vi "save program.vi"(8 "error in (no error)":errorcluster, 10 "Array":T1=[{"Action"=enum."Start", "Angle Min [°]"=0.0, "Angle Max [°]"=0.0, "Torque Min [oz-in]"=0.0, "Torque Max [oz-in]"=0.0}, {"Action"=enum."Return to Home", "Angle Min [°]"=0.0, "Angle Max [°]"=0.0, "Torque Min [oz-in]"=0.0, "Torque Max [oz-in]"=0.0}, {"Action"=enum."End", "Angle Min [°]"=0.0, "Angle Max [°]"=0.0, "Torque Min [oz-in]"=0.0, "Torque Max [oz-in]"=0.0}], 11 "Programs in":refnum<class "Programs.lvclass">) -> (0 "error out":errorcluster, 3 "Programs out":refnum<class "Programs.lvclass">)   [LabVIEW 2025, in "Programs.lvclass"]
uses:
  Programs.lvclass
  Programs.lvclass/Programs.ctl
  <vilib>/JDP Science/JSONtext/JSONtext.lvlib
  Controls/Sequencer/action enum.ctl
  Controls/Sequencer/step cluster.ctl
  Controls/Sequencer/sequence array.ctl
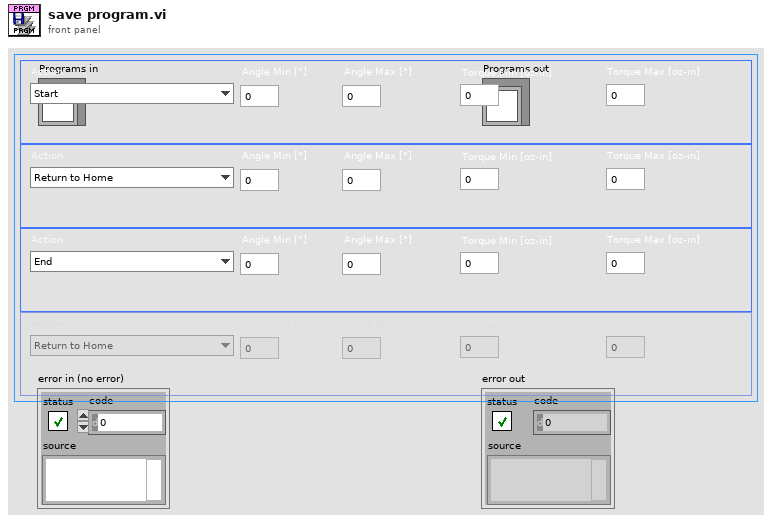
[diagram p1: front panel]
types:
  T1 = typedef "sequence array.ctl" = T2[]
  T2 = typedef "step cluster.ctl" = cluster{"Action":T3, "Angle Min [°]":dbl, "Angle Max [°]":dbl, "Torque Min [oz-in]":dbl, "Torque Max [oz-in]":dbl}
  T3 = typedef "action enum.ctl" = enum16{"Start", "Angle", "Return to Home", "End"}
  T4 = enum16{"open", "replace", "create", "open or create", "replace or create", "replace or create with confirmation"}
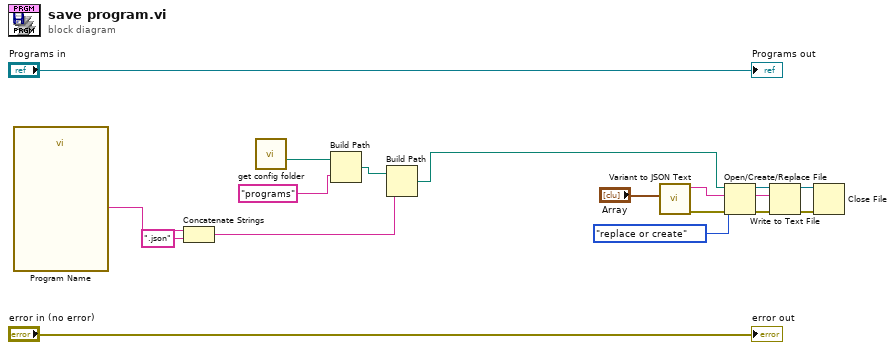
[diagram p0: block diagram]
diagram:
  n1 = call "Program Name"() -> ("Part Number"=w6:string)  [unwired: 17 in, 2 out]
  n2 = Concatenate Strings(w6, ".json" ("string")) -> (w3:string)
  n3 = call "get config folder.vi"() -> ("Config folder path"=w8:path)  [unwired: 11 in]
  n4 = Build Path(base path=w8, name or relative path="programs") -> (appended path=w4:path)
  n5 = Build Path(base path=w4, name or relative path=w3) -> (appended path=w2:path)
  n6 = call <vilib>:"Variant to JSON Text.vi"("Variant"="Array") -> ("error out"=w9:errorcluster, "<JSON>"=w10:string)  [unwired: 8 in, 1 out]
  n7 = Open/Create/Replace File(file path (use dialog)=w2, error in=w9, operation (0:open)=T4."replace or create") -> (refnum out=w13:refnum<file>, error out=w12:errorcluster)  [unwired: 3 in, 1 out]
  n8 = Write to Text File(file (use dialog)=w13, text=w10, error in=w12) -> (refnum out=w14:refnum<file>, error out=w15:errorcluster)  [unwired: 1 in, 1 out]
  n9 = Close File(refnum=w14, error in=w15) -> ()  [unwired: 2 out]
  "error out" <- "error in (no error)"
  "Programs out" <- "Programs in"
